vi "DVR Q Create Async.vi"() -> ()   [LabVIEW 2021, in "Q Async.lvlib"]
uses:
  Q Async.lvlib
  DVR Q Loop.vi
panel:
  in  "Numeric":i32=4
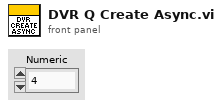
[diagram p1: front panel]
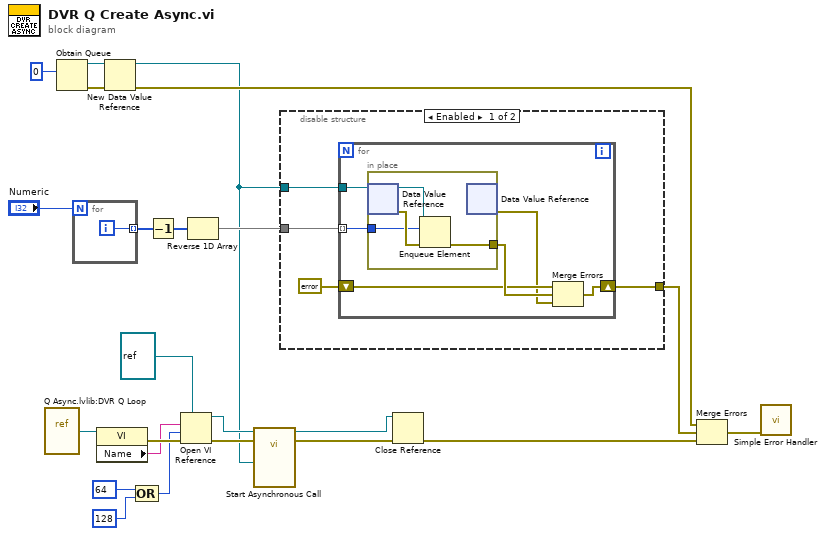
[diagram p0: block diagram]
diagram:
  n1 = vi-ref "Q Async.lvlib:DVR Q Loop.vi"() -> (w12:refnum<vi>)
  n2 = Obtain Queue(element data type=0) -> (queue out=w20:refnum<queue>, error out=w17:errorcluster)  [unwired: 4 in, 1 out]
  n3 = for {
    N: "Numeric" -> [_]
    tunnel: [w24] -> w22 mode=indexing
    i -> [w24]
  }
  n4 = property class="VI"(reference=w12) -> (error out=w11:errorcluster, "Name"=w10:string)  [unwired: 1 in, 1 out]
  n5 = New Data Value Reference(data value=w20, error in=w17) -> (data value reference=w4:refnum<data-value>, error out=w14:errorcluster)
  n6 = Compound Arithmetic op=OR(64 ("options"), 128 ("options")) -> (w7:i32)
  n7 = Decrement(x=w22) -> (x-1=w23:i32[])
  n8 = Open VI Reference(type specifier VI Refnum (for type only)=refnum<vi> refnum, vi path=w10, options=w7, error in (no error)=w11) -> (vi reference=w5:refnum<vi>, error out=w6:errorcluster)  [unwired: 2 in]
  n9 = Reverse 1D Array(array=w23) -> (reversed array=w18:i32[])
  n10 = call-by-ref "Start Asynchronous Call"(reference=w5, error in=w6, "DVR"=w4) -> (reference out=w3:refnum<vi>, error out=w2:errorcluster)  [unwired: 11 in]
  n11 = disable-structure shown="Enabled" {
    disable-tunnel: w18 -> [w28 _]
    disable-tunnel: [w26 _] -> w16
    disable-tunnel: w4 -> [w25 _]
    frame Enabled {
      n12 = for {
        tunnel: w25 -> [w34]
        tunnel: w28 -> [w33] mode=indexing
        shift-right: [w31] -> w26
        shift-left: errorcluster {"status"=FALSE, "code"=0, "source"=""} ("error out") -> [w30]
        n13 = in-place {
          in-place-border: w33 -> [w35]
          in-place-border: [w36] -> w32
          n14 = in-place-dvr #1(w34) -> (w38:refnum<queue>, w37:errorcluster)
          n15 = Enqueue Element(queue=w38, element=w35, error in (no error)=w37) -> (error out=w36:errorcluster)  [unwired: 1 in, 2 out]
          n16 = in-place-dvr #1() -> (w29:errorcluster)  [unwired: 1 in, 1 out]
        }
        n17 = Merge Errors(w30, w32, w29) -> (w31:errorcluster)
      }
    }
    frame Disabled {
    }
  }
  n18 = Close Reference(reference=w3, error in (no error)=w2) -> (error out=w1:errorcluster)
  n19 = Merge Errors(w14, w16, w1) -> (w15:errorcluster)
  n20 = call <vilib>:"Simple Error Handler.vi"("error in (no error)"=w15) -> ()  [unwired: 4 in, 5 out]
